vi "Sift Alice's Key.vi"(8 "error in":errorcluster, 10 "Alice's Raw Data in":u8[](array[numeric]), 11 "Bob's Data in":u32[](array[numeric])) -> (0 "error out":errorcluster, 1 "Incorrect Bob's data":bool, 2 "Bob's correct measurements indexes":u32[](array[numeric]))   [LabVIEW 2018]
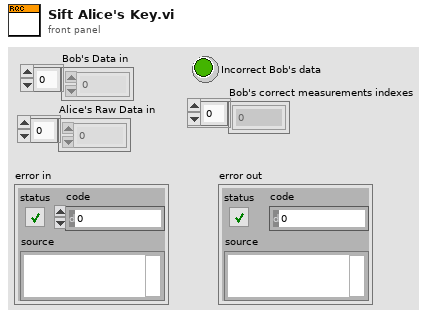
[diagram p1: front panel]
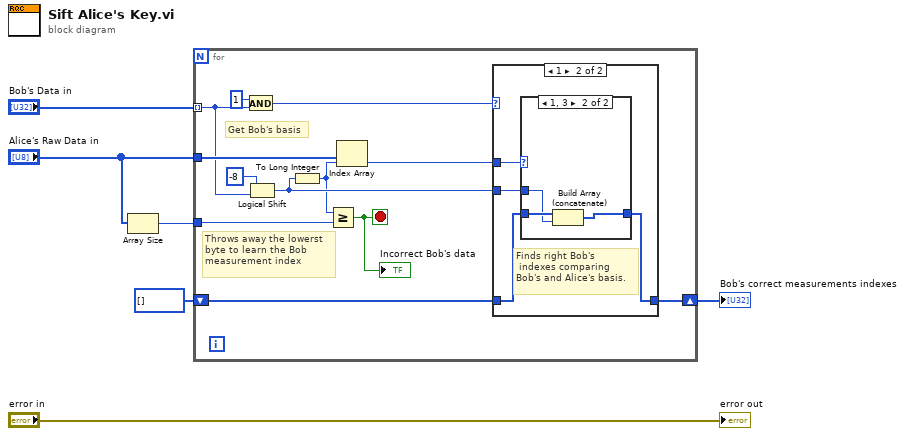
[diagram p0: block diagram]
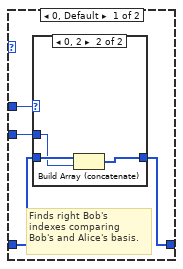
[diagram p2: hidden frame]
diagram:
  n1 = Array Size(array="Alice's Raw Data in") -> (size(s)=w4:i32)
  n2 = for {
    tunnel: "Bob's Data in" -> [w16] mode=indexing
    tunnel: "Alice's Raw Data in" -> [w17]
    shift-right: [w12] -> w6
    shift-left: u32[] [] -> [w13]
    tunnel: w4 -> [w10]
    stop <- w8 stop-if-true
    # "Get Bob's basis"
    # "Throws away the lowerst\nbyte to learn the Bob\nmeasurement index"
    n3 = And(x=u32 1, y=w16) -> (x .and. y?=w7:u32)
    n4 = Logical Shift(y=-8, x=w16) -> (x << y=w11:u32)
    n5 = To Long Integer(number=w11) -> (32bit integer=w9:i32)
    n6 = Greater Or Equal?(x=w9, y=w10) -> (x >= y?=w8:bool)
    "Incorrect Bob's data" <- w8
    n7 = Index Array(array=w17, index=w9) -> (element=w14:u8)
    n8 = case shown="1" w7 {
      tunnel: w14 -> [w19 w27]
      tunnel: w13 -> [w22 w28]
      tunnel: [w21 w30] -> w12
      tunnel: w11 -> [w20 w29]
      frame 0, Default {
        # "Finds right Bob's \nindexes comparing \nBob's and Alice's basis."
        n9 = case shown="0, 2" w19 {
          tunnel: w22 -> [w23 w26]
          tunnel: [w23 w25] -> w21
          tunnel: w20 -> [_ w24]
          frame 1, Default {
          }
          frame 0, 2 {
            n10 = Build Array (concatenate)(w26, w24) -> (w25:u32[])
          }
        }
      }
      frame 1 {
        # "Finds right Bob's\n indexes comparing\nBob's and Alice's basis."
        n11 = case shown="1, 3" w27 {
          tunnel: w28 -> [w31 w34]
          tunnel: [w31 w33] -> w30
          tunnel: w29 -> [_ w32]
          frame 0, Default {
          }
          frame 1, 3 {
            n12 = Build Array (concatenate)(w34, w32) -> (w33:u32[])
          }
        }
      }
    }
  }
  "Bob's correct measurements indexes" <- w6
  "error out" <- "error in"
